vi "ActFollowTrajectoryCommon.vi"(6 "End Orientation":dbl, 7 "Orientation":T1, 9 "currentPose":T2={"TRANSLATION"={"X"=0.0, "Y"=0.0}, "ROTATION"={"VALUE"=0.0, "COS"=1.0, "SIN"=0.0}} {"ROTATION"."SIN" format="%13.4f"; "ROTATION"."COS" format="%13.4f"; "ROTATION"."VALUE" format="%13.4f"; "TRANSLATION"."Y" format="%14.3f"; "TRANSLATION"."X" format="%14.3f"}, 10 "Trajectory":T5 {"States"."POSE"."ROTATION"."SIN" format="%13.4f"; "States"."POSE"."ROTATION"."COS" format="%13.4f"; "States"."POSE"."ROTATION"."VALUE" format="%13.4f"; "States"."POSE"."TRANSLATION"."Y" format="%14.3f"; "States"."POSE"."TRANSLATION"."X" format="%14.3f"; "TotalTImeSecs" format="%20.3f"}, 11 "FirstTime":bool) -> (0 "Done":bool, 1 "vAngularDemand":dbl, 2 "vYSpeedDemand":dbl, 3 "vXSpeedDemand":dbl)   [LabVIEW 2023]
uses:
  <vilib>/Rock Robotics/WPI/ThirdParty/JAS_Junk/TrajLib/TypeDef/TRAJECTORY.ctl
  <vilib>/Rock Robotics/WPI/ThirdParty/JAS_Junk/TrajLib/TypeDef/TRAJ_STATE.ctl
  <vilib>/Rock Robotics/WPI/ThirdParty/JAS_Junk/TrajLib/TypeDef/POSE2D.ctl
  <vilib>/Rock Robotics/WPI/ThirdParty/JAS_Junk/TrajLib/TypeDef/TRANSLATION2D.ctl
  <vilib>/Rock Robotics/WPI/ThirdParty/JAS_Junk/TrajLib/TypeDef/ROTATION2D.ctl
  Autonomous/TrajectoryOrientation.ctl
  <vilib>/Rock Robotics/WPI/ThirdParty/JAS_Junk/TrajLib/VI/Util_GetTime_U32.vi
  <vilib>/Rock Robotics/WPI/ThirdParty/JAS_Junk/TrajLib/HolDrvCtrl_New.vi
  <vilib>/Rock Robotics/WPI/ThirdParty/JAS_Junk/TrajLib/HolDrvCtrl_PackPID.vi
  <vilib>/Rock Robotics/WPI/ThirdParty/JAS_Junk/TrajLib/HolDrvCtrl_SetTolerance.vi
  <vilib>/Rock Robotics/WPI/ThirdParty/JAS_Junk/TrajLib/HolDrvCtrl_SetEnabled.vi
  <vilib>/Rock Robotics/WPI/ThirdParty/JAS_Junk/TrajLib/HolDrvCtrl_Calculate_Trajectory.vi
  <vilib>/Rock Robotics/WPI/ThirdParty/JAS_Junk/TrajLib/HolDrvCtrl_AtReference.vi
  <vilib>/Rock Robotics/WPI/ThirdParty/JAS_Junk/TrajLib/ProfiledPIDController_NewPeriod.vi
  <vilib>/Rock Robotics/WPI/ThirdParty/JAS_Junk/TrajLib/ProfiledPIDController_SetIntegratorRange.vi
  <vilib>/Rock Robotics/WPI/ThirdParty/JAS_Junk/TrajLib/ProfiledPIDController_DisableContInput.vi
  <vilib>/Rock Robotics/WPI/ThirdParty/JAS_Junk/TrajLib/ProfiledPIDController_EnableContInput.vi
  <vilib>/Rock Robotics/WPI/ThirdParty/JAS_Junk/TrajLib/TrapProfConstraint_New.vi
  <vilib>/Rock Robotics/WPI/ThirdParty/JAS_Junk/TrajLib/MathUtil_Clamp.vi
  <vilib>/Rock Robotics/WPI/ThirdParty/JAS_Junk/TrajLib/Conv_Deg_Radians.vi
  <vilib>/Rock Robotics/WPI/ThirdParty/JAS_Junk/TrajLib/Rotation2d_CreateAngle.vi
  <vilib>/Rock Robotics/WPI/ThirdParty/JAS_Junk/TrajLib/PIDController_NewPeriod.vi
  <vilib>/Rock Robotics/WPI/ThirdParty/JAS_Junk/TrajLib/PIDController_SetIntegratorRange.vi
  <vilib>/Rock Robotics/WPI/ThirdParty/JAS_Junk/TrajLib/PIDController_Reset.vi
  <vilib>/Rock Robotics/WPI/ThirdParty/JAS_Junk/TrajLib/HolDrvCtrl_Calculate.vi
  <vilib>/Rock Robotics/WPI/ThirdParty/JAS_Junk/TrajLib/Pose2d_getXYAngle.vi
  <vilib>/Rock Robotics/WPI/ThirdParty/JAS_Junk/TrajLib/Rotation2d_GetRadians.vi
  <vilib>/Rock Robotics/WPI/ThirdParty/JAS_Junk/TrajLib/TrapProfState_New.vi
  <vilib>/Rock Robotics/SystemInterfaces/NetworkCommunication/NetComm_UsageReport_report.vi
  <vilib>/Rock Robotics/WPI/ThirdParty/JAS_Junk/TrajLib/PIDController_DisableContinousInput.vi
  <vilib>/Rock Robotics/WPI/ThirdParty/JAS_Junk/TrajLib/PIDController_EnableContinousInput.vi
  <vilib>/Rock Robotics/WPI/ThirdParty/JAS_Junk/TrajLib/Rotation2d_GetAngleCosSin.vi
  <vilib>/Rock Robotics/WPI/ThirdParty/JAS_Junk/TrajLib/Pose2d_RelativeTo.vi
  <vilib>/Rock Robotics/WPI/ThirdParty/JAS_Junk/TrajLib/Pose2d_getRotation.vi
  <vilib>/Rock Robotics/WPI/ThirdParty/JAS_Junk/TrajLib/Rotation2d_Minus.vi
  <vilib>/Rock Robotics/WPI/ThirdParty/JAS_Junk/TrajLib/ProfiledPIDController_Calculate_Meas_Goal.vi
  <vilib>/Rock Robotics/WPI/ThirdParty/JAS_Junk/TrajLib/PIDController_Calculate_SP_PV.vi
  <vilib>/Rock Robotics/WPI/ThirdParty/JAS_Junk/TrajLib/ProfiledPIDController_Reset_PosOnly.vi
  <vilib>/Rock Robotics/WPI/ThirdParty/JAS_Junk/TrajLib/ChassisSpeeds_FromFieldRelativeSpeeds.vi
  <vilib>/Rock Robotics/WPI/ThirdParty/JAS_Junk/TrajLib/Transform2d_Create_PosePose.vi
  <vilib>/Rock Robotics/WPI/ThirdParty/JAS_Junk/TrajLib/Pose2d_New_TRRO.vi
  <vilib>/Rock Robotics/WPI/ThirdParty/JAS_Junk/TrajLib/Rotation2d_UnaryMinus.vi
  <vilib>/Rock Robotics/WPI/ThirdParty/JAS_Junk/TrajLib/Rotation2d_RotateBy.vi
  <vilib>/Rock Robotics/WPI/ThirdParty/JAS_Junk/TrajLib/ProfiledPIDController_SetGoal_PosOnly.vi
  <vilib>/Rock Robotics/WPI/ThirdParty/JAS_Junk/TrajLib/ProfiledPIDController_Calculate_Meas.vi
  <vilib>/Rock Robotics/WPI/ThirdParty/JAS_Junk/TrajLib/PIDController_SetSetpoint.vi
  <vilib>/Rock Robotics/WPI/ThirdParty/JAS_Junk/TrajLib/PIDController_Calculate_PV.vi
  <vilib>/Rock Robotics/WPI/ThirdParty/JAS_Junk/TrajLib/ProfiledPIDController_Reset.vi
  <vilib>/Rock Robotics/WPI/ThirdParty/JAS_Junk/TrajLib/Rotation2d_GetCos.vi
  <vilib>/Rock Robotics/WPI/ThirdParty/JAS_Junk/TrajLib/Rotation2d_GetSin.vi
  <vilib>/Rock Robotics/WPI/ThirdParty/JAS_Junk/TrajLib/ChassisSpeeds_New.vi
  <vilib>/Rock Robotics/WPI/ThirdParty/JAS_Junk/TrajLib/Translation2d_RotateBy.vi
  <vilib>/Rock Robotics/WPI/ThirdParty/JAS_Junk/TrajLib/Translation2d_Minus.vi
  <vilib>/Rock Robotics/WPI/ThirdParty/JAS_Junk/TrajLib/Rotation2d_CreateXY.vi
  <vilib>/Rock Robotics/WPI/ThirdParty/JAS_Junk/TrajLib/ProfiledPIDController_SetGoal.vi
  <vilib>/Rock Robotics/WPI/ThirdParty/JAS_Junk/TrajLib/TrapProfile_New.vi
  <vilib>/Rock Robotics/WPI/ThirdParty/JAS_Junk/TrajLib/ProfiledPIDController_GetPeriod.vi
  <vilib>/Rock Robotics/WPI/ThirdParty/JAS_Junk/TrajLib/TrapProfile_Calculate.vi
  <vilib>/Rock Robotics/WPI/ThirdParty/JAS_Junk/TrajLib/ControllerUtil_GetModulusError.vi
  <vilib>/Rock Robotics/WPI/ThirdParty/JAS_Junk/TrajLib/Translation2d_Create.vi
  <vilib>/Rock Robotics/WPI/ThirdParty/JAS_Junk/TrajLib/Util_CalcDist.vi
  <vilib>/Rock Robotics/WPI/ThirdParty/JAS_Junk/TrajLib/TrapProfile_ShouldFlipAcceleration.vi
  <vilib>/Rock Robotics/WPI/ThirdParty/JAS_Junk/TrajLib/TrapProfile_Direct.vi
  <vilib>/Rock Robotics/WPI/ThirdParty/JAS_Junk/TrajLib/PIDController_GetPeriod.vi
  <vilib>/Rock Robotics/SystemInterfaces/Utilities/FPGA_UtilitiesRead LocalTime.vi
  <vilib>/Rock Robotics/WPI/ThirdParty/JAS_Junk/TrajLib/VI/Util_GetTime_U64.vi
  <vilib>/Rock Robotics/WPI/ThirdParty/JAS_Junk/TrajLib/Globals/Util_LibraryGlobals.vi
  <vilib>/Rock Robotics/Network Tables/NT Write Number.vi
  Drive/DriveGlobal.vi
  <vilib>/Rock Robotics/WPI/ThirdParty/JAS_Junk/TrajLib/Trajectory_Library.lvlib
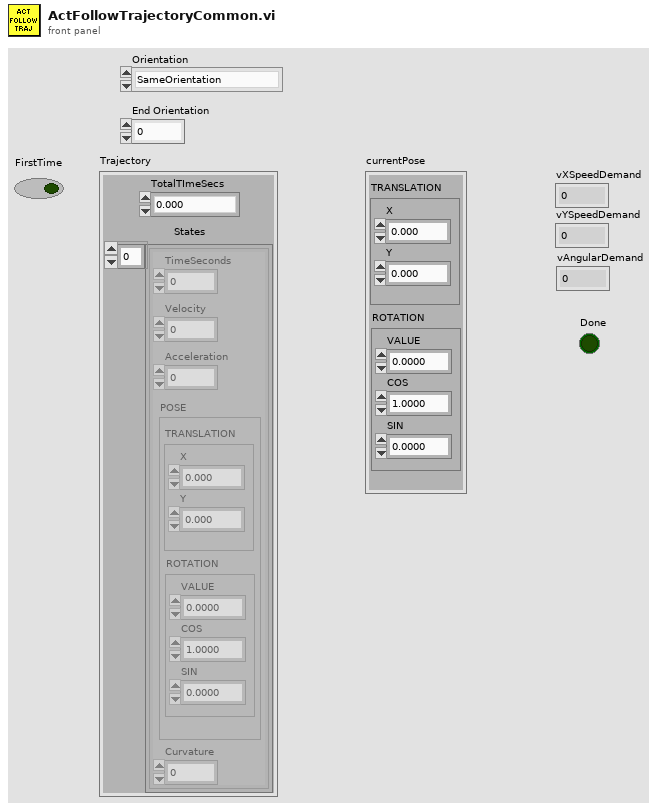
[diagram p1: front panel]
types:
  T1 = typedef "TrajectoryOrientation.ctl" = enum16{"SameOrientation", "RotateToEndOrientation"}
  T2 = typedef "Trajectory_Library.lvlib/POSE2D.ctl" = cluster{"TRANSLATION":T3, "ROTATION":T4}
  T3 = typedef "Trajectory_Library.lvlib/TRANSLATION2D.ctl" = cluster{"X":dbl, "Y":dbl}
  T4 = typedef "Trajectory_Library.lvlib/ROTATION2D.ctl" = cluster{"VALUE":dbl, "COS":dbl, "SIN":dbl}
  T5 = typedef "Trajectory_Library.lvlib/TRAJECTORY.ctl" = cluster{"TotalTImeSecs":dbl, "States":T6[]}
  T6 = typedef "Trajectory_Library.lvlib/TRAJ_STATE.ctl" = cluster{"TimeSeconds":dbl, "Velocity":dbl, "Acceleration":dbl, "POSE":T2, "Curvature":dbl}
  T7 = typedef "Trajectory_Library.lvlib/PID_TUNING.ctl" = cluster{"Kp":dbl, "Ki":dbl, "Kd":dbl, "MaximumIntegral":dbl, "MinimumIntegral":dbl, "IntegralZone":dbl}
  T8 = typedef "Trajectory_Library.lvlib/PROFILED_PID_CONTROLLER.ctl" = cluster{"Controller":T9, "Goal":T10, "Setpoint":T10, "Constraint":T11}
  T9 = typedef "Trajectory_Library.lvlib/PID_CONTROLLER.ctl" = cluster{"Kp":dbl, "Ki":dbl, "Kd":dbl, "Period":dbl, "Max_Integral":dbl, "Min_Integral":dbl, "Max_Input":dbl, "Min_Input":dbl, "Continuous":bool, "PositionError":dbl, "VelocityError":dbl, "PrevError":dbl, "Total_Integral":dbl, "PositionTolerance":dbl, "VelocityTolerance":dbl, "SetPoint":dbl, "Kf":dbl, "Prev_Deriv":dbl, "Prev_Deriv 2":dbl, "DerivativeFilter":bool, "Min_Output":dbl, "Max_Output":dbl, "Prev_F_P":dbl, "Prev_F_P_2":dbl, "AntiWindupActive":bool, "Measurement":dbl, "IntegralZone":dbl}
  T10 = typedef "Trajectory_Library.lvlib/TRAPEZOID_PROFILE_STATE.ctl" = cluster{"Position":dbl, "Velocity":dbl}
  T11 = typedef "Trajectory_Library.lvlib/TRAPEZOID_PROFILE_CONSTRAINT.ctl" = cluster{"MaxVelocity":dbl, "MaxAcceleration":dbl}
  T12 = typedef "Trajectory_Library.lvlib/HOLONOMIC_PACK_TUNING.ctl" = cluster{"X PID Tuning":T7, "Y PID Tuning":T7, "thetaProfiledPID_CTRL":T8}
  T13 = typedef "Trajectory_Library.lvlib/CHASSIS_SPEEDS.ctl" = cluster{"vX":dbl, "vY":dbl, "vOmega":dbl}
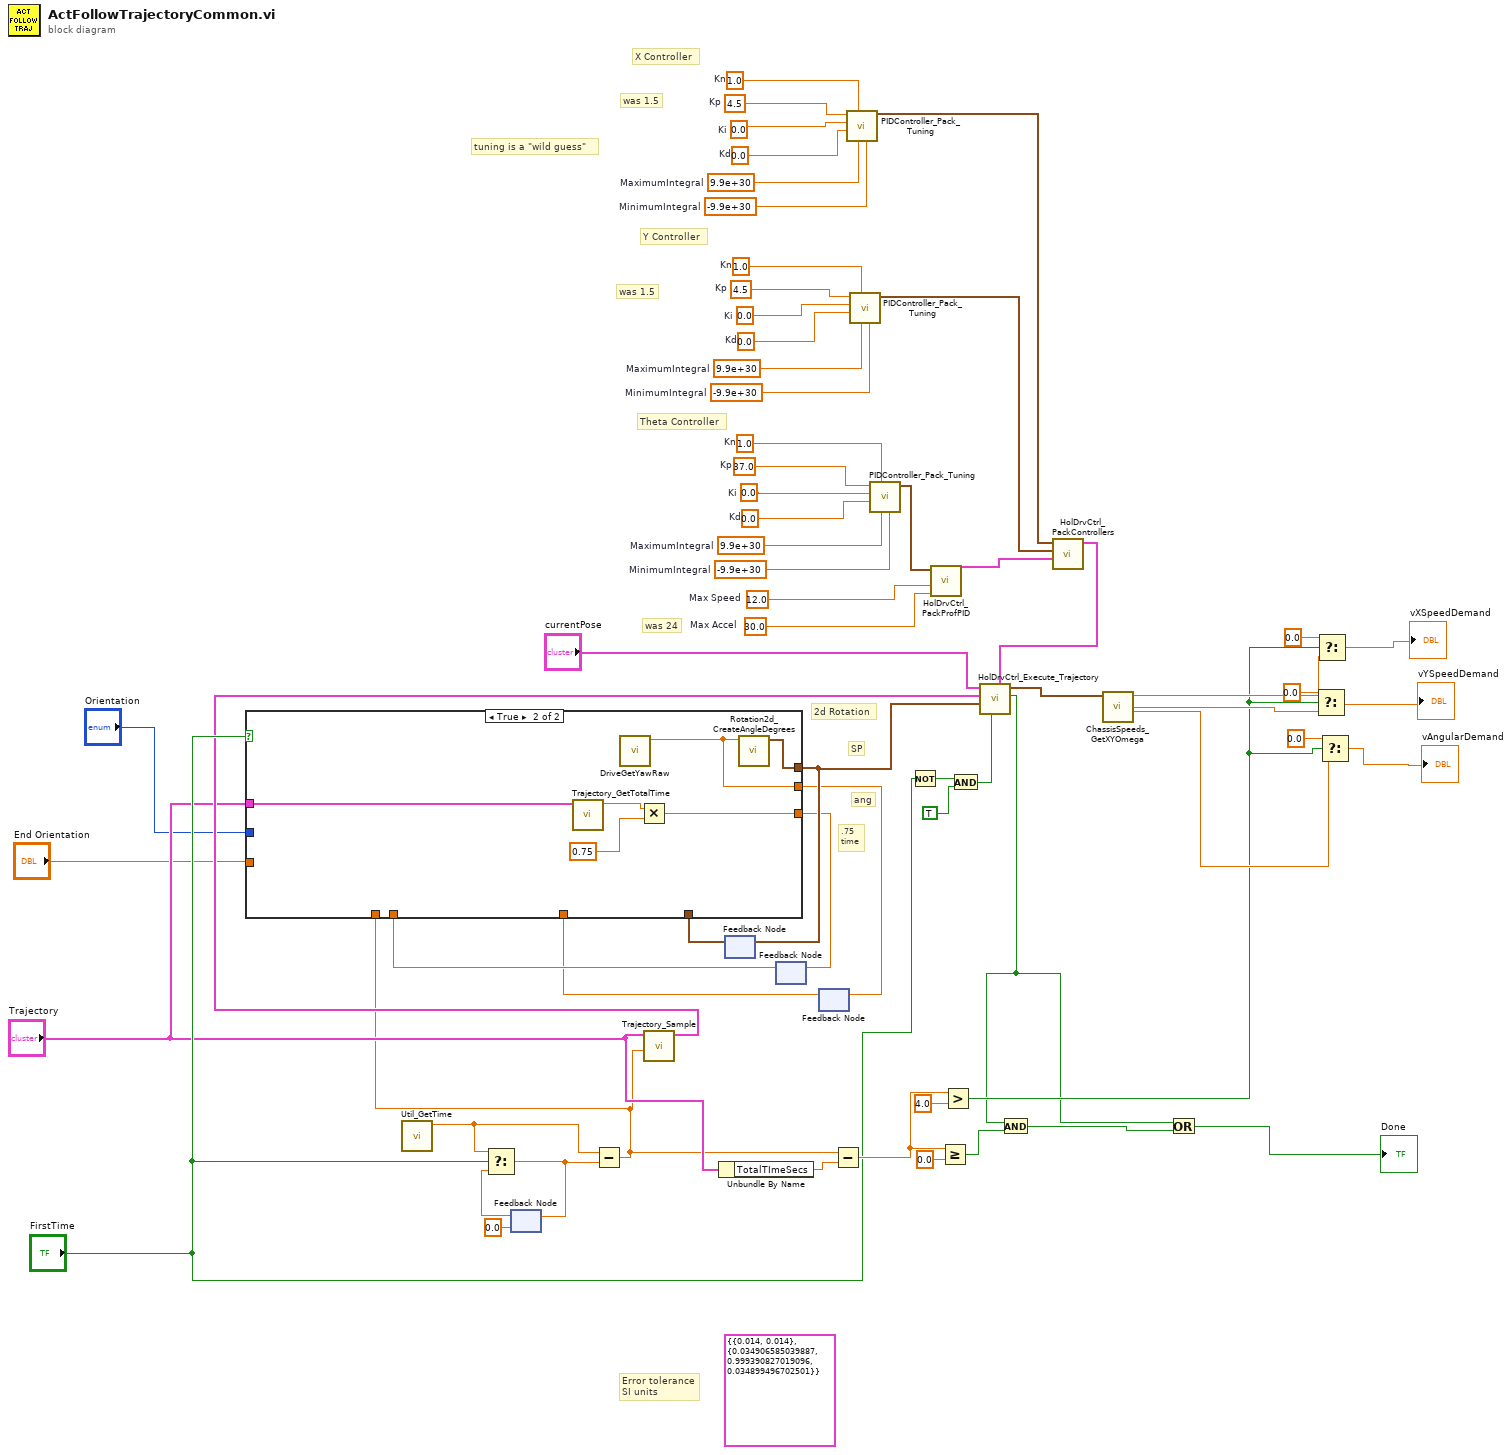
[diagram p0: block diagram]
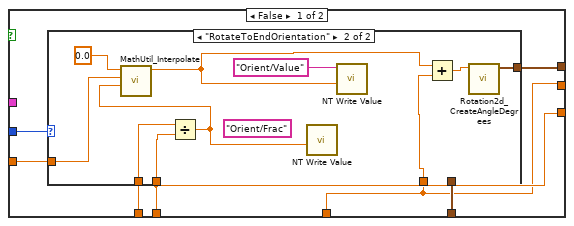
[diagram p2: hidden frame]
diagram:
  (unwired) T2 {"TRANSLATION"={"X"=0.014, "Y"=0.014}, "ROTATION"={"VALUE"=0.034906585039887, "COS"=0.999390827019096, "SIN"=0.034899496702501}} ("Tolerance")
  w39 = 1.0  # Kn
  w42 = 37.0  # Kp
  w51 = 0.0  # Ki
  w52 = 0.0  # Kd
  w53 = 9.9e+30  # MaximumIntegral
  w54 = -9.9e+30  # MinimumIntegral
  w37 = 1.0  # Kn
  w40 = 4.5  # Kp
  w43 = 0.0  # Ki
  w44 = 0.0  # Kd
  w45 = 9.9e+30  # MaximumIntegral
  w46 = -9.9e+30  # MinimumIntegral
  w38 = 1.0  # Kn
  w41 = 4.5  # Kp
  w47 = 0.0  # Ki
  w48 = 0.0  # Kd
  w49 = 9.9e+30  # MaximumIntegral
  w50 = -9.9e+30  # MinimumIntegral
  w36 = 30.0  # Max Accel
  w35 = 12.0  # Max Speed
  # ".75\ntime"
  # "ang"
  # "was 24"
  # "SP"
  # "Error tolerance\nSI units"
  # "was 1.5"
  # "was 1.5"
  # "tuning is a \"wild guess\""
  # "2d Rotation"
  # "Theta Controller"
  # "Y Controller"
  # "X Controller"
  n1 = call <vilib>:"Util_GetTime.vi"() -> ("FPGA_Time_Seconds"=w62:dbl)  [unwired: 9 in, 2 out]
  n2 = feedback #1(0.0) -> (w64:dbl)
  n3 = Select(t=w62, s="FirstTime", f=w64) -> (s? t:f=w61:dbl)
  n4 = feedback-in #1(w61) -> ()
  n5 = Subtract(x=w62, y=w61) -> (x-y=w13:dbl)
  n6 = call <vilib>:"Trajectory_Sample.vi"("Time"=w13, "InputTRAJECTORY"="Trajectory") -> ("OutputTRAJ_STATE"=w19:T6)  [unwired: 9 in]
  n7 = Unbundle By Name("Trajectory") -> ("TotalTImeSecs"=w60:dbl)
  n8 = feedback #2() -> (w20:T4)  [unwired: 1 in]
  n9 = feedback #3() -> (w16:dbl)  [unwired: 1 in]
  n10 = feedback #4() -> (w11:dbl)  [unwired: 1 in]
  n11 = case shown="True" "FirstTime" {
    tunnel: [w69 w88] -> w21
    tunnel: w20 -> [w70 _]
    tunnel: "Trajectory" -> [_ w87]
    tunnel: [w66 w84] -> w17
    tunnel: w16 -> [w66 _]
    tunnel: "Orientation" -> [w71 _]
    tunnel: "End Orientation" -> [w68 _]
    tunnel: w13 -> [w67 _]
    tunnel: [w65 w83] -> w12
    tunnel: w11 -> [w65 _]
    frame False {
      n12 = case shown="\"RotateToEndOrientation\"" w71 {
        tunnel: w70 -> [w72 _]
        tunnel: [w72 w76] -> w69
        tunnel: w68 -> [_ w81]
        tunnel: w67 -> [_ w80]
        tunnel: w66 -> [_ w79]
        tunnel: w65 -> [_ w78]
        frame "SameOrientation", Default {
        }
        frame "RotateToEndOrientation" {
          (unwired) "Orient/Frac" ("name")
          n13 = Divide(x=w80, y=w79) -> (x/y=w73:dbl)
          n14 = call <vilib>:"MathUtil_Interpolate.vi"("T"=w73, "EndValue"=w81, "StartValue"=0.0) -> ("InterpolatedValue"=w74:dbl)  [unwired: 8 in]
          n15 = call-poly <vilib>:"NT Write Value.vi"("value"=w73) -> ()  [unwired: 10 in, 1 out]
          n16 = call-poly <vilib>:"NT Write Value.vi"("value"=w74, "name"="Orient/Value") -> ()  [unwired: 9 in, 1 out]
          n17 = Add(x=w74, y=w78) -> (x+y=w77:dbl)
          n18 = call <vilib>:"Rotation2d_CreateAngleDegrees.vi"("Angle_Degrees"=w77) -> ("ROTATION"=w76:T4)  [unwired: 10 in]
        }
      }
    }
    frame True {
      n19 = call <vilib>:"Trajectory_GetTotalTime.vi"("TRAJECTORY"=w87) -> ("TotalTime_Sec"=w86:dbl)  [unwired: 10 in]
      n20 = call "DriveGetYawRaw.vi"() -> ("YawRaw"=w83:dbl)  [unwired: 11 in]
      n21 = Multiply(x=w86, y=0.75) -> (x*y=w84:dbl)
      n22 = call <vilib>:"Rotation2d_CreateAngleDegrees.vi"("Angle_Degrees"=w83) -> ("ROTATION"=w88:T4)  [unwired: 10 in]
    }
  }
  n23 = feedback-in #2(w21) -> ()
  n24 = feedback-in #3(w17) -> ()
  n25 = feedback-in #4(w12) -> ()
  n26 = Subtract(x=w13, y=w60) -> (x-y=w57:dbl)
  n27 = call <vilib>:"PIDController_Pack_Tuning.vi"("MinimumIntegral"=w46, "MaximumIntegral"=w45, "Kn"=w37, "Kd"=w44, "Ki"=w43, "Kp"=w40) -> ("PID Tuning"=w9:T7)  [unwired: 5 in]
  n28 = call <vilib>:"PIDController_Pack_Tuning.vi"("MinimumIntegral"=w50, "MaximumIntegral"=w49, "Kn"=w38, "Kd"=w48, "Ki"=w47, "Kp"=w41) -> ("PID Tuning"=w8:T7)  [unwired: 5 in]
  n29 = call <vilib>:"PIDController_Pack_Tuning.vi"("MinimumIntegral"=w54, "MaximumIntegral"=w53, "Kn"=w39, "Kd"=w52, "Ki"=w51, "Kp"=w42) -> ("PID Tuning"=w34:T7)  [unwired: 5 in]
  n30 = Not(x="FirstTime") -> (.not. x?=w24:bool)
  n31 = call <vilib>:"HolDrvCtrl_PackProfPID.vi"("Max Accel"=w36, "Max Speed"=w35, "Theta PID Tuning"=w34) -> ("Theta PID CONTROLLER"=w7:T8)  [unwired: 8 in]
  n32 = Greater Or Equal?(x=w57, y=0.0) -> (x >= y?=w4:bool)
  n33 = Greater?(x=w57, y=4.0) -> (0:w25:bool)
  n34 = And(x=w24, y=TRUE ("Enabled")) -> (x .and. y?=w5:bool)
  n35 = call <vilib>:"HolDrvCtrl_PackControllers.vi"("thetaProfiledPID_CTRL"=w7, "Y PID Tuning"=w8, "X PID Tuning"=w9) -> ("HOLONOMIC_CTRL_PACK_TUNING"=w10:T12)  [unwired: 8 in]
  n36 = call <vilib>:"HolDrvCtrl_Execute_Trajectory.vi"("HOLONOMIC_CTRL_PACK_TUNING"=w10, "Reset"=w5, "angleRef"=w21, "desiredTrajState"=w19, "currentPose"="currentPose") -> ("AtReference"=w2:bool, "calcChassisSpeed"=w6:T13)  [unwired: 4 in, 1 out]
  n37 = And(x=w2, y=w4) -> (x .and. y?=w3:bool)
  n38 = call <vilib>:"ChassisSpeeds_GetXYOmega.vi"("CHASSIS"=w6) -> ("vAngular"=w27:dbl, "vY"=w29:dbl, "vX"=w31:dbl)  [unwired: 8 in]
  n39 = Or(x=w2, y=w3) -> (x .or. y?=→"Done":bool)
  n40 = Select(t=0.0, s=w25, f=w29) -> (s? t:f=→"vYSpeedDemand":dbl)
  n41 = Select(t=0.0, s=w25, f=w31) -> (s? t:f=→"vXSpeedDemand":dbl)
  n42 = Select(t=0.0, s=w25, f=w27) -> (s? t:f=→"vAngularDemand":dbl)
